vi "Connection_Management_Test.vi"() -> ()   [LabVIEW 2017]
uses:
  Classes/ADCP.lvclass
panel:
  in  "ADCP Session Parameters":T1
  in  "ADCP in":refnum<class "ADCP.lvclass">
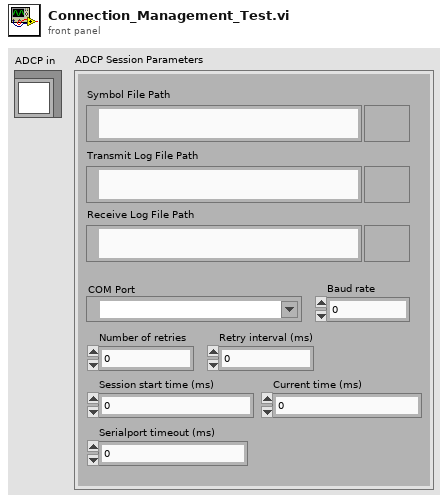
[diagram p1: front panel]
types:
  T1 = cluster{"Symbol File Path":path, "Transmit Log File Path":path, "Receive Log File Path":path, "COM Port":refnum<visa-resource-name>, "Baud rate":u32, "Number of retries":u16, "Retry interval (ms)":u16, "Session start time (ms)":u32, "Current time (ms)":u32, "Serialport timeout (ms)":u32}
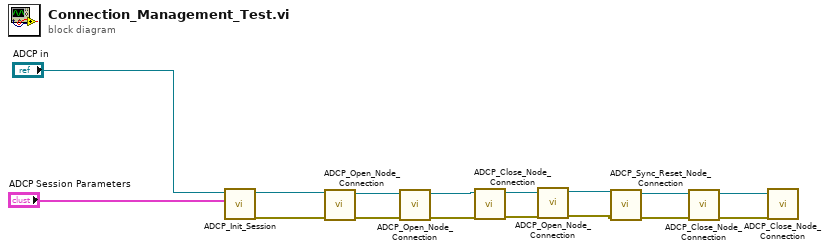
[diagram p0: block diagram]
diagram:
  n1 = call "ADCP_Init_Session.vi"("ADCP Session Parameters"="ADCP Session Parameters", "ADCP in"="ADCP in") -> ("error out"=w13:errorcluster, "ADCP out"=w14:refnum<class "ADCP.lvclass">)  [unwired: 8 in]
  n2 = call "ADCP_Open_Node_Connection.vi"("error in (no error)"=w13, "ADCP In"=w14) -> ("error out"=w11:errorcluster, "ADCP Out"=w12:refnum<class "ADCP.lvclass">)  [unwired: 8 in]
  n3 = call "ADCP_Open_Node_Connection.vi"("error in (no error)"=w11, "ADCP In"=w12) -> ("error out"=w9:errorcluster, "ADCP Out"=w10:refnum<class "ADCP.lvclass">)  [unwired: 8 in]
  n4 = call "ADCP_Close_Node_Connection.vi"("error in (no error)"=w9, "ADCP In"=w10) -> ("error out"=w7:errorcluster, "ADCP Out"=w8:refnum<class "ADCP.lvclass">)  [unwired: 8 in]
  n5 = call "ADCP_Open_Node_Connection.vi"("error in (no error)"=w7, "ADCP In"=w8) -> ("error out"=w5:errorcluster, "ADCP Out"=w6:refnum<class "ADCP.lvclass">)  [unwired: 8 in]
  n6 = call "ADCP_Sync_Reset_Node_Connection.vi"("error in (no error)"=w5, "ADCP In"=w6) -> ("error out"=w3:errorcluster, "ADCP Out"=w4:refnum<class "ADCP.lvclass">)  [unwired: 8 in]
  n7 = call "ADCP_Close_Node_Connection.vi"("error in (no error)"=w3, "ADCP In"=w4) -> ("error out"=w1:errorcluster, "ADCP Out"=w2:refnum<class "ADCP.lvclass">)  [unwired: 8 in]
  n8 = call "ADCP_Close_Node_Connection.vi"("error in (no error)"=w1, "ADCP In"=w2) -> ()  [unwired: 8 in, 2 out]
